vi "Do.vi"(8 "error in (no error)":errorcluster, 10 "Actor in":refnum<class "Actor.lvclass">, 11 "Draw Assert Data Msg":refnum<class "Draw Assert Data Msg.lvclass">) -> (0 "error out":errorcluster, 2 "Actor out":refnum<class "Actor.lvclass">)   [LabVIEW 2016, in "UserInterface.lvlib" / "Draw Assert Data Msg.lvclass"]
doc: "This VI delivers the message to the actor by calling the appropriate method(s) on the actor."
uses:
  Draw Assert Data Msg.lvclass
  <vilib>/ActorFramework/Actor/Actor.lvclass
  UserInterface/UserInterface.lvclass
  C:/Program Files/National Instruments/LabVIEW 2016/vi.lib/ActorFramework/Actor/Actor.lvclass
  Draw Assert Data Msg.lvclass/Draw Assert Data Msg.ctl
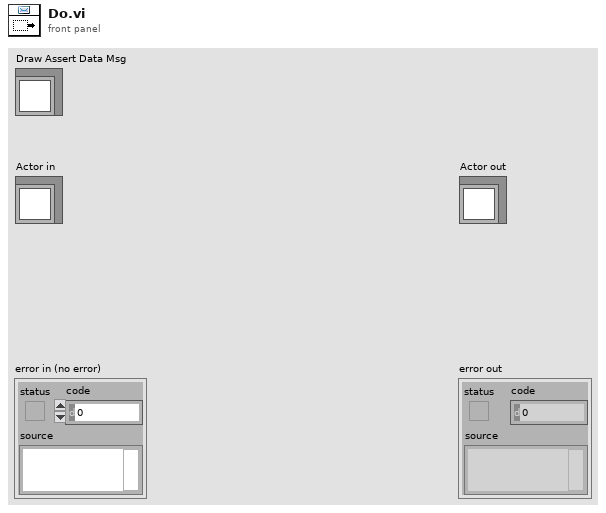
[diagram p1: front panel]
types:
  T1 = typedef "UserInterface.lvlib/UserInterface.lvclass/Sort Configuration.ctl" = cluster{"Column to Sort By":u32, "Order":enum16{"ascending", "descending"}}
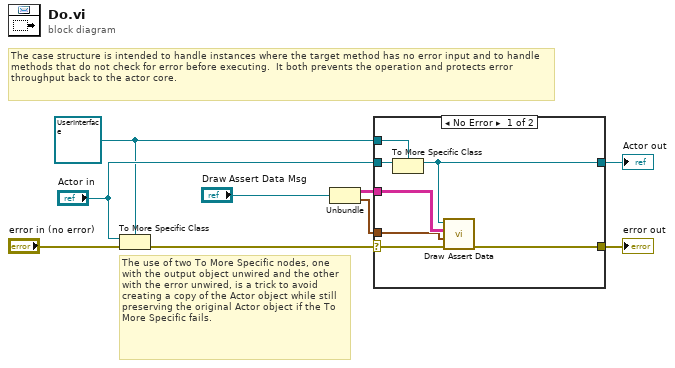
[diagram p0: block diagram]
diagram:
  w3 = refnum<class "UserInterface.lvclass"> refnum ("Actor in")
  # "The use of two To More Specific nodes, one with the output object unwired and the other with the error unwired, is a trick to avoid creating a copy of the Actor object while still preserving the original Actor object if the To More Specific fails."
  # "The case structure is intended to handle instances where the target method has no error input and to handle methods that do not check for error before executing.  It both prevents the operation and protects error throughput back to the actor core."
  n1 = To More Specific Class(target class=w3, reference="Actor in", error in="error in (no error)") -> (error out=w7:errorcluster)  [unwired: 1 out]
  n2 = Unbundle("Draw Assert Data Msg") -> (w2:string[][], w1:T1)
  n3 = case shown="No Error" w7 {
    selector: w7 -> [w15 w18]
    tunnel: [w16 w18] -> w6
    tunnel: [w12 w17] -> w5
    tunnel: "Actor in" -> [w14 w17]
    tunnel: w3 -> [w13 _]
    tunnel: w2 -> [w11 _]
    tunnel: w1 -> [w10 _]
    frame No Error {
      n4 = To More Specific Class(target class=w13, reference=w14) -> (specific class reference=w12:refnum<class "UserInterface.lvclass">)  [unwired: 1 in, 1 out]
      n5 = call "Draw Assert Data.vi"("error in (no error)"=w15, "Sort Configuration"=w10, "Assert Data"=w11, "UserInterface in"=w12) -> ("error out"=w16:errorcluster)  [unwired: 7 in]
    }
    frame Error {
      # "If type check fails, pass the original object out again."
    }
  }
  "error out" <- w6
  "Actor out" <- w5
